vi "Stop Core.vi"(10 "final error code":i32, 11 "UDP_Service in":refnum<class "UDP_Service.lvclass">) -> (3 "UDP_Service out":refnum<class "UDP_Service.lvclass">)   [LabVIEW 2016, in "CoreAssertAPI.lvlib" / "UDP_Service.lvclass"]
doc: "(<B>Filename</B>: Actor Framework.lvlib:Actor.lvclass:Stop Core.vi)\n\nDefines what the actor does before it stops. Use the <B>final error code</B> input to determine whether the actor shut down in response to an error.\n\nBy default, this method does nothing. A descendant class may override it to define behavior, such as shutting down any processes the actor initiated in its override of the Actor Core method."
uses:
  UDP_Service.lvclass
  UDP_Service.lvclass/UDP_Service.ctl
  <vilib>/ActorFramework/Actor/Actor.lvclass
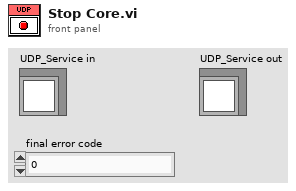
[diagram p1: front panel]
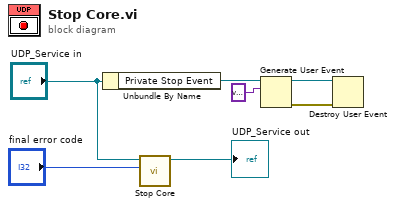
[diagram p0: block diagram]
diagram:
  n1 = Unbundle By Name("UDP_Service in") -> ("Private Stop Event"=w4:refnum<user-event>)
  n2 = call-parent "Stop Core.vi"("final error code"="final error code", "Actor in"="UDP_Service in") -> ("Actor out"=→"UDP_Service out":refnum<class "UDP_Service.lvclass">)  [unwired: 9 in]
  n3 = Generate User Event(user event=w4, event data cluster=variant ("event data")) -> (user event out=w3:refnum<user-event>, error out=w2:errorcluster)  [unwired: 2 in]
  n4 = Destroy User Event(user event=w3, error in=w2) -> ()  [unwired: 1 out]
